vi "Read Real Time Eye.vi"(8 "error in (no error)":errorcluster, 10 "Waveform Source (0: Channel 1)":i32(ring) items=["Channel 1", "Channel 2", "Channel 3", "Channel 4", "Common 1", "Common 2", "Differential 1", "Differential 2", "Memory 1", "Memory 2", "Memory 3", "Memory 4", "Function 1", "Function 2", "Function 3", "Function 4", "Function 5", "Function 6", "Function 7", "Function 8", "Function 9", "Function 10", "Function 11", "Function 12", "Function 13", "Function 14", "Function 15", "Function 16"], 11 "VISA resource name":refnum<visa-resource-name>) -> (0 "error out":errorcluster, 1 "Unit Interval":dbl, 2 "Waveform Number":dbl, 3 "VISA resource name out":refnum<visa-resource-name>)   [LabVIEW 2020, in "Agilent 90000 Series.lvlib"]
doc: "Queries the number of waveforms and unit intervals in the real time eye.\n\n<b>Notes:</b> \n1. This VI is new in firmware version 5.00. \n2. Make sure the waveform source is on before querying."
uses:
  Agilent 90000 Series.lvlib
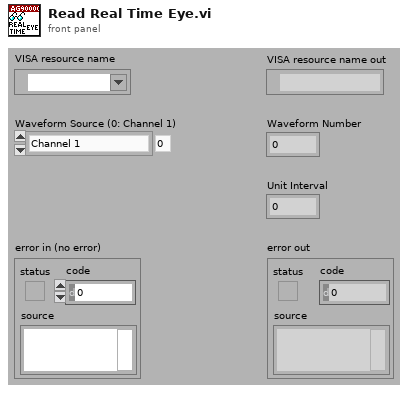
[diagram p1: front panel]
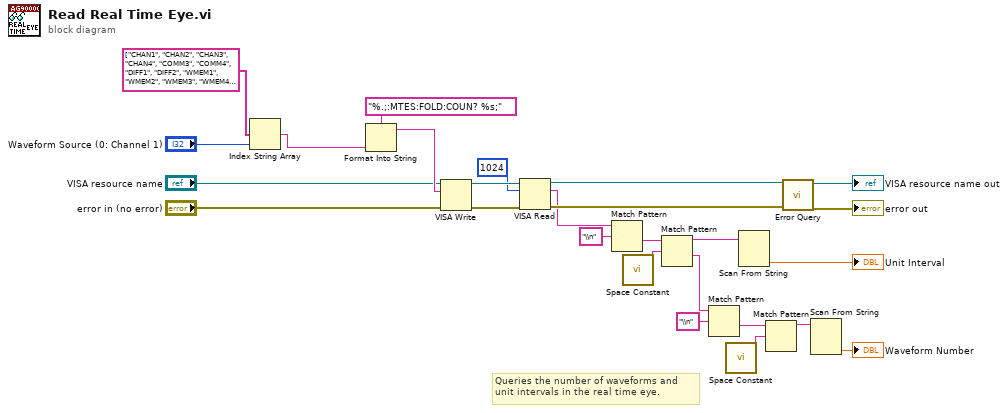
[diagram p0: block diagram]
diagram:
  # "Queries the number of waveforms and\nunit intervals in the real time eye."
  n1 = Index String Array(1:"Waveform Source (0: Channel 1)", 2:string[] ["CHAN1", "CHAN2", "CHAN3", "CHAN4", "COMM3", "COMM4", "DIFF1", "DIFF2", "WMEM1", "WMEM2", "WMEM3", "WMEM4", "FUNC1", "FUNC2", "FUNC3", "FUNC4", "FUNC5", "FUNC6", "FUNC7", "FUNC8", "FUNC9", "FUNC10", "FUNC11", "FUNC12", "FUNC13", "FUNC14", "FUNC15", "FUNC16"] ("string array")) -> (0:w18:string)  [unwired: 1 in]
  n2 = Format Into String(format string="%.;:MTES:FOLD:COUN? %s;", w18) -> (resulting string=w25:string)  [unwired: 2 in, 1 out]
  n3 = VISA Write(VISA resource name="VISA resource name", write buffer=w25, error in (no error)="error in (no error)") -> (VISA resource name out=w17:refnum<visa-resource-name>, error out=w16:errorcluster)  [unwired: 1 out]
  n4 = VISA Read(VISA resource name=w17, byte count=u32 1024, error in (no error)=w16) -> (VISA resource name out=w14:refnum<visa-resource-name>, read buffer=w5:string, error out=w13:errorcluster)  [unwired: 1 out]
  n5 = Match Pattern(string=w5, regular expression="\\n") -> (after substring=w11:string)  [unwired: 1 in, 3 out]
  n6 = call <vilib>:"Space Constant.vi"() -> ("String"=w10:string)
  n7 = Match Pattern(string=w11, regular expression=w10) -> (before substring=w4:string, after substring=w9:string)  [unwired: 1 in, 2 out]
  n8 = Match Pattern(string=w9, regular expression="\\n") -> (after substring=w7:string)  [unwired: 1 in, 3 out]
  n9 = call <vilib>:"Space Constant.vi"() -> ("String"=w6:string)
  n10 = Scan From String(input string=w4) -> (output 1=→"Unit Interval":dbl)  [unwired: 4 in, 3 out]
  n11 = Match Pattern(string=w7, regular expression=w6) -> (before substring=w2:string)  [unwired: 1 in, 3 out]
  n12 = call "Error Query.vi"("error in (no error)"=w13, "VISA resource name"=w14) -> ("error out"=→"error out":errorcluster, "VISA resource name out"=→"VISA resource name out":refnum<visa-resource-name>)  [unwired: 6 in, 2 out]
  n13 = Scan From String(input string=w2) -> (output 1=→"Waveform Number":dbl)  [unwired: 4 in, 3 out]
